vi "Main Page.vi"(8 "error in (no error)":errorcluster, 11 "Node Ptr":T6 format="%.0x") -> (0 "error out":errorcluster)   [LabVIEW 2021, in "Modbus Master System Explorer.lvlib"]
uses:
  Modbus Master System Explorer.lvlib
  <vilib>/NI VeriStand/Custom Device API/Custom Device Item Ref.ctl
  Shared/Controls/Interface Type.ctl
  Shared/Controls/Parity.ctl
  Shared/Controls/Serial Type.ctl
  Shared/Controls/Flow Control.ctl
  Shared/Write Mode.ctl
  Shared/Constants.vi
  <vilib>/NI VeriStand/Custom Device API/Set Item Property (U16).vi
  <vilib>/NI VeriStand/Custom Device API/Custom Device API.lvlib
  Shared/Modbus Master Shared.lvlib
panel:
  in  "Write Refresh Rate (ms)":i32
  in  "Write Mode":T1
  in  "WebBrowser":refnum<k7>(container)
  in  "Maximum Channels per Read":i32
  in  "Read Refresh Rate (ms)":i32
  in  "Export to Kepware Server":bool
  in  "Name":string
  in  "Master Settings Tabs":enum32{"TCP Master", "Serial Master"}(tab)
  in  "Timeout (ms)":i32
  in  "Address":string
  in  "Port":u16
  in  "Baud Rate":string(combo)
  out "Data Bits":u32=7
  in  "VISA resource name":refnum<visa-resource-name>
  in  "flow control (none)":T2 items=["None", "XON/XOFF", "RTS/CTS", "XON/XOFF & RTS/CTS", "DTR/DSR", "XON/XOFF & DTR/DSR"]
  in  "parity (even)":T3=2 items=["None", "Odd", "Even", "Mark", "Space"]
  in  "serial type":T4
  out "Stop Bits":u32
  in  "Wire Mode":i16(ring)=-2 items=["Non-NI RS485"=-2, "Unknown"=-1, "RS485/Wire4"=0, "RS485/Wire2-EchoDTR"=1, "RS485/Wire2-CtrlDTR"=2, "RS485/Wire2-Auto"=3, "RS232/DTE"=128, "RS232/DCE"=129, "RS232/AUTO"=130]
  in  "Interface Type":T5
  in  "Header":cluster{"Section Name":string}={"Section Name"="Modbus Master to Slave Settings"}
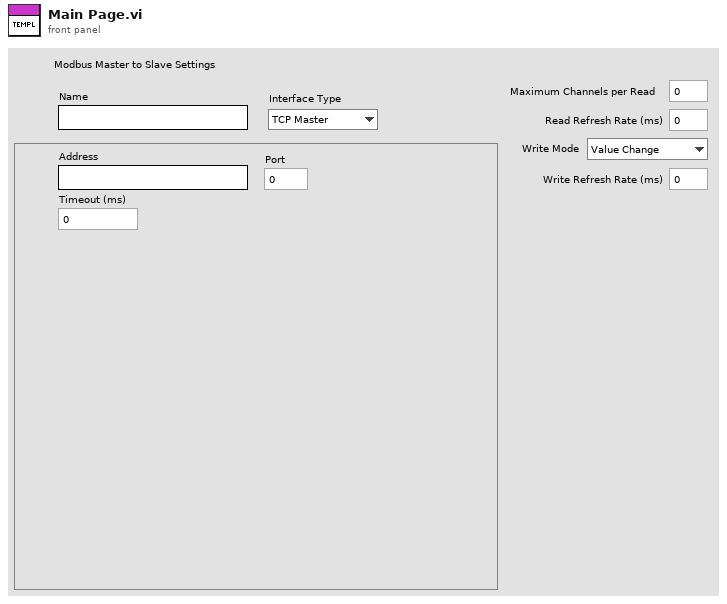
[diagram p1: front panel]
types:
  T1 = typedef "Modbus Master Shared.lvlib/Write Mode.ctl" = enum16{"Value Change", "Interval"}
  T2 = typedef "Modbus Master Shared.lvlib/Flow Control.ctl" = u16
  T3 = typedef "Modbus Master Shared.lvlib/Parity.ctl" = u16
  T4 = typedef "Modbus Master Shared.lvlib/Serial Type.ctl" = enum16{"RTU", "ASCII"}
  T5 = typedef "Modbus Master Shared.lvlib/Interface Type.ctl" = enum16{"TCP Master", "Serial Master", "TCP Slave", "Serial Slave"}
  T6 = typedef "Custom Device API.lvlib/Custom Device Item Ref.ctl" = u64
  T7 = enum8{"Enabled", "Disabled", "Disabled and Grayed Out"}
  T8 = typedef "Custom Device API.lvlib/Custom Device Commands.ctl" = enum16{"Default", "Item renamed", "Shutdown", "Dynamic button pressed"}
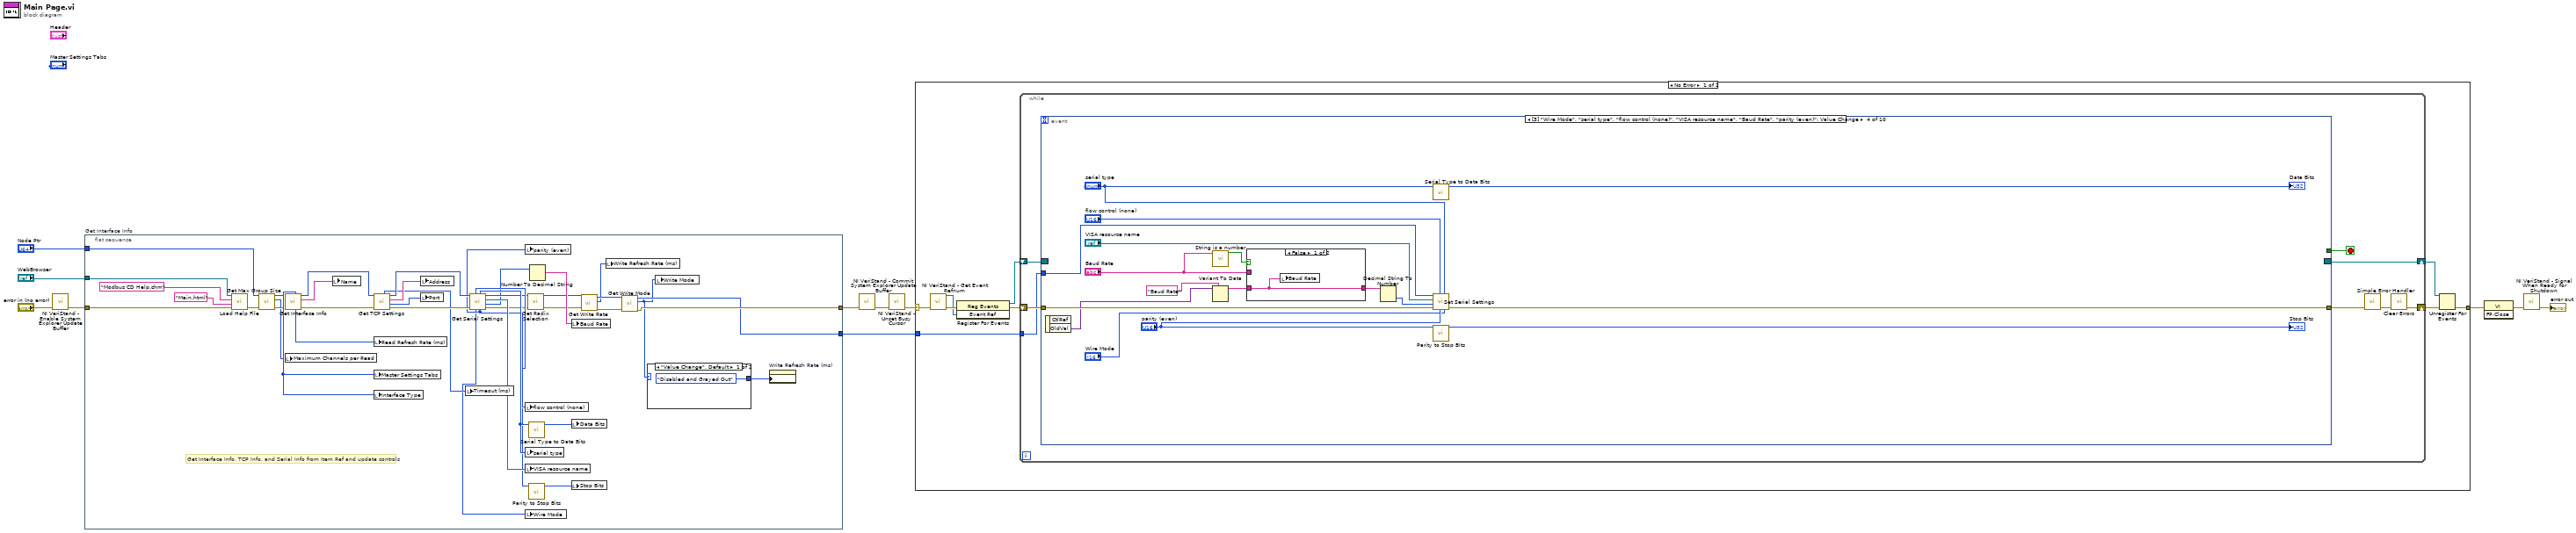
[diagram p0: block diagram]
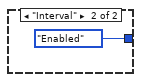
[diagram p2: hidden frame]
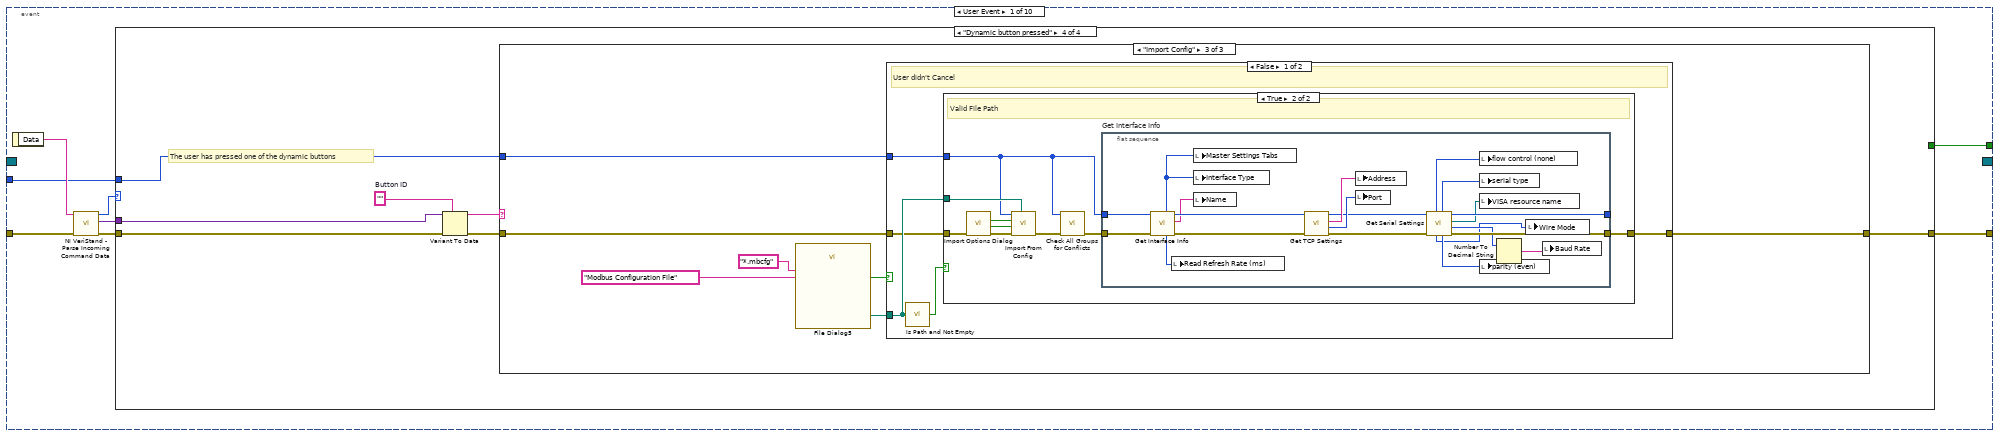
[diagram p3: hidden frame]
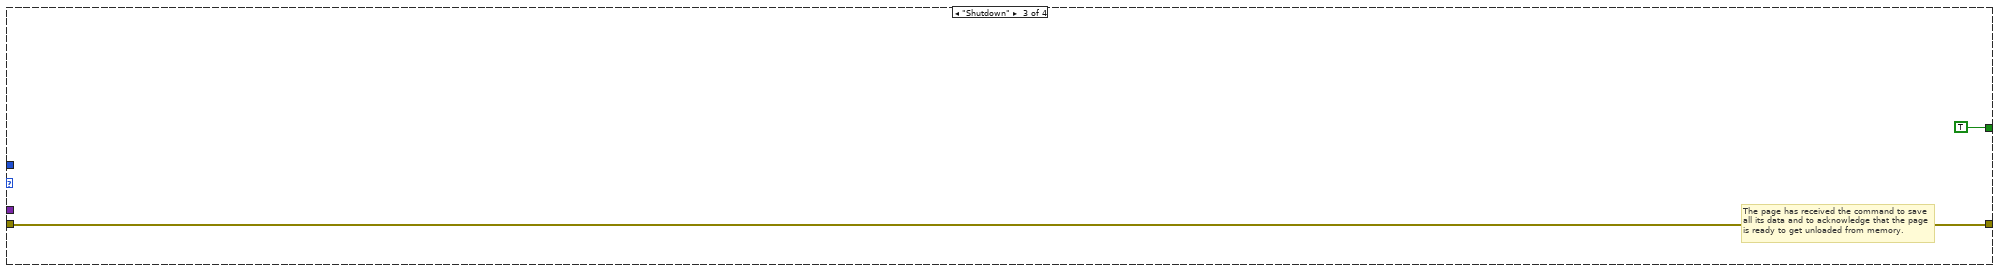
[diagram p6: hidden frame]
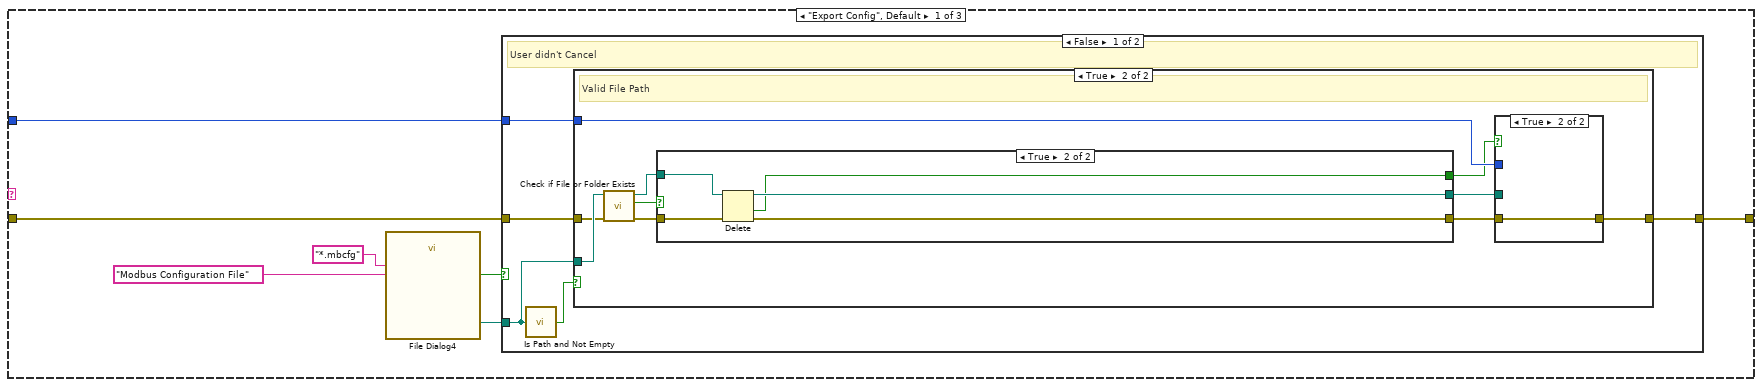
[diagram p7: hidden frame]
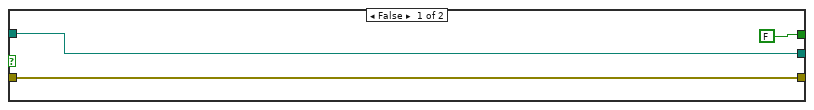
[diagram p9: hidden frame]
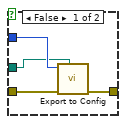
[diagram p10: hidden frame]
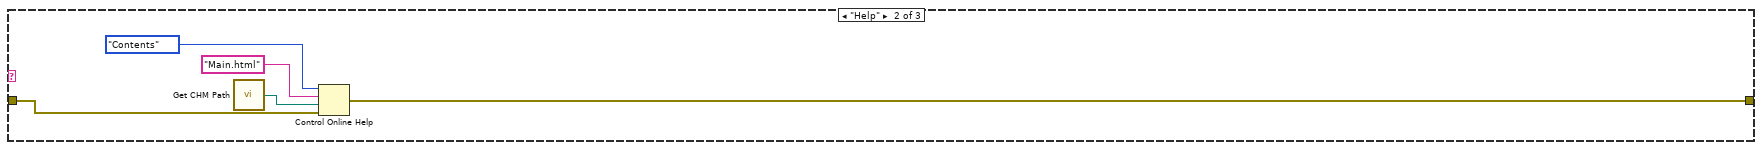
[diagram p12: hidden frame]
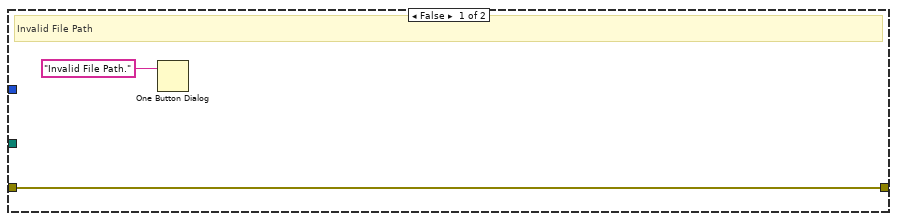
[diagram p13: hidden frame]
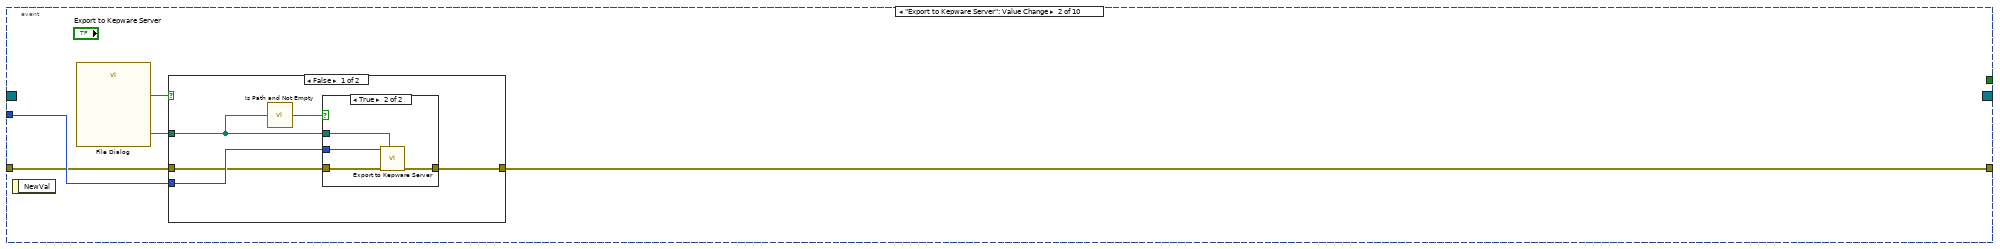
[diagram p15: hidden frame]
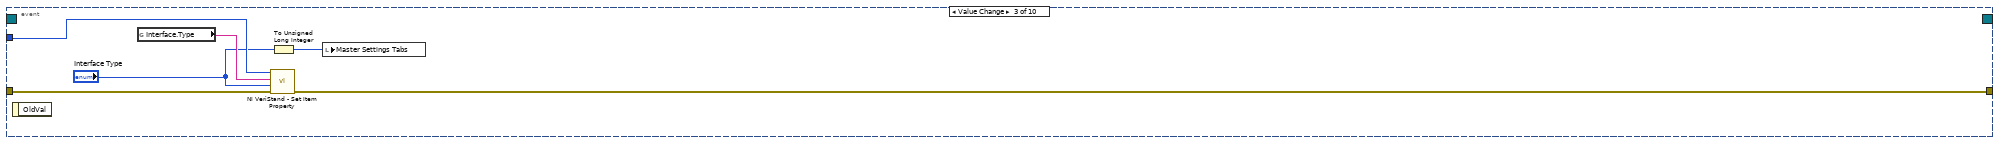
[diagram p18: hidden frame]
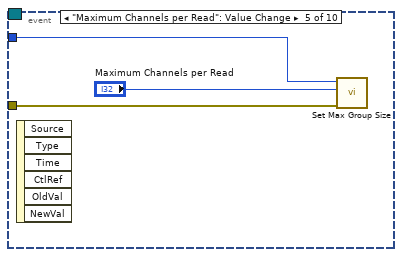
[diagram p20: hidden frame]
diagram:
  n1 = call <vilib>:"NI VeriStand - Enable System Explorer Update Buffer.vi"("error in (no error)"="error in (no error)") -> ("error out"=w1:errorcluster)  [unwired: 10 in]
  n2 = flat-sequence "Get Interface Info" {
    tunnel: w1 -> [w23]
    tunnel: "Node Ptr" -> [w35]
    tunnel: [w18] -> w4
    tunnel: [w15] -> w6
    tunnel: "WebBrowser" -> [w26]
    frame #0 {
      # "Get Interface Info, TCP Info, and Serial Info from Item Ref and update controls"
      n3 = call "Load Help File.vi"("error in (no error)"=w23, "HTML File"="Main.html", "Main CHM File"="Modbus CD Help.chm", "SHDocVw.IWebBrowser2"=w26) -> ("error out"=w22:errorcluster)  [unwired: 7 in]
      n4 = call "Get Max Group Size.vi"("error in (no error)"=w22, "Item Ref in"=w35) -> ("error out"=w33:errorcluster, "Value"=w32:i32, "Item Ref out"=w34:T6)  [unwired: 7 in]
      n5 = local write "Maximum Channels per Read"(w32) -> ()
      n6 = call "Get Interface Info.vi"("error in (no error)"=w33, "Device Item Ref in"=w34) -> ("error out"=w43:errorcluster, "Name"=w41:string, "Item Ref out"=w44:T6, "Refresh Rate"=w40:i32, "Interface Type"=w42:T5)  [unwired: 4 in, 1 out]
      n7 = local write "Name"(w41) -> ()
      n8 = call "Get TCP Settings.vi"("error in (no error)"=w43, "Item Ref in"=w44) -> ("error out"=w48:errorcluster, "Port"=w49:u16, "Address"=w50:string, "Item Ref out"=w47:T6, "Timeout"=w31:i32)  [unwired: 5 in]
      n9 = local write "Read Refresh Rate (ms)"(w40) -> ()
      n10 = local write "Master Settings Tabs"(w42) -> ()
      n11 = local write "Interface Type"(w42) -> ()
      n12 = local write "Address"(w50) -> ()
      n13 = local write "Port"(w49) -> ()
      n14 = local write "Timeout (ms)"(w31) -> ()
      n15 = call "Get Serial Settings.vi"("error in (no error)"=w48, "Item Ref in"=w47) -> ("error out"=w30:errorcluster, "baud rate"=w28:u32, "VISA resource name"=w45:refnum<visa-resource-name>, "Item Ref out"=w29:T6, "parity (even)"=w37:T3, "serial type"=w38:T4, "Wire Mode"=w21:i32, "flow control (none)"=w46:T2)  [unwired: 2 in]
      n16 = local write "parity (even)"(w37) -> ()
      n17 = local write "flow control (none)"(w46) -> ()
      n18 = local write "serial type"(w38) -> ()
      n19 = local write "VISA resource name"(w45) -> ()
      n20 = local write "Wire Mode"(w21) -> ()
      n21 = call "Get Radix Selection.vi"("error in (no error)"=w30, "Item Ref in"=w29) -> ("error out"=w20:errorcluster, "Item Ref out"=w17:T6)  [unwired: 7 in, 1 out]
      n22 = call "Serial Type to Data Bits.vi"("serial type"=w38) -> ("Data Bits"=w39:u32)  [unwired: 10 in]
      n23 = call "Parity to Stop Bits.vi"("parity"=w37) -> ("Stop Bits"=w36:u32)  [unwired: 10 in]
      n24 = Number To Decimal String(number=w28) -> (decimal integer string=w27:string)  [unwired: 1 in]
      n25 = local write "Baud Rate"(w27) -> ()
      n26 = local write "Data Bits"(w39) -> ()
      n27 = local write "Stop Bits"(w36) -> ()
      n28 = call "Get Write Rate.vi"("error in (no error)"=w20, "Item Ref in"=w17) -> ("error out"=w19:errorcluster, "Value"=w14:i32, "Item Ref out"=w16:T6)  [unwired: 7 in]
      n29 = local write "Write Refresh Rate (ms)"(w14) -> ()
      n30 = call "Get Write Mode.vi"("error in (no error)"=w19, "Item Ref in"=w16) -> ("error out"=w18:errorcluster, "Write Mode"=w12:T1, "Item Ref out"=w15:T6)  [unwired: 7 in]
      n31 = case shown="\"Value Change\", Default" w12 {
        tunnel: [T7."Disabled and Grayed Out" ("Disabled") T7."Enabled" ("Disabled")] -> w13
        frame "Value Change", Default {
        }
        frame "Interval" {
        }
      }
      n32 = local write "Write Mode"(w12) -> ()
      n33 = property on="Write Refresh Rate (ms)" class="DigNum (strict)"("DisabledEnum"=w13) -> ()  [unwired: 2 in, 2 out]
    }
  }
  n34 = call <vilib>:"NI VeriStand - Commit System Explorer Update Buffer.vi"("error in (no error)"=w4) -> ("error out"=w3:errorcluster)  [unwired: 10 in]
  n35 = call <vilib>:"NI VeriStand - Unset Busy Cursor.vi"("error in (no error)"=w3) -> ("error out"=w7:errorcluster)  [unwired: 10 out]
  n36 = case shown="No Error" w7 {
    selector: w7 -> [w53 w256]
    tunnel: [w58 w254] -> w11
    tunnel: w6 -> [w54 _]
    frame No Error {
      n37 = call <vilib>:"NI VeriStand - Get Event Refnum.vi"("error in (no error)"=w53) -> ("error out"=w61:errorcluster, "Event Ref"=w57:refnum<user-event>)  [unwired: 9 out]
      n38 = register-events(error in=w61, w57) -> (reference out=w55:refnum<event-registration>, error out=w56:errorcluster)  [unwired: 1 in]
      n39 = while {
        tunnel: w54 -> [w65]
        shift-right: [w62] -> w59
        shift-left: w56 -> [w68]
        shift-right: [w69] -> w60
        shift-left: w55 -> [w67]
        stop <- w66 stop-if-true
        n40 = event shown="[3] \"Wire Mode\", \"serial type\", \"flow control (none)\", \"VISA resource name\", \"Baud Rate\", \"parity (even)\": Value Change" {
          selector: w67 -> [_ _ _ _ _ _ _ _ _ _]
          dyn-events: [_ _ _ _ _ _ _ _ _ _] -> w69
          timeout: _ -> [_ _ _ _ _ _ _ _ _ _]
          tunnel: w68 -> [w77 w176 w194 w211 w216 w220 w225 w230 w234 w241]
          tunnel: [w73 _ _ _ _ _ _ _ _ _] -> w66
          tunnel: [w72 w175 w191 w209 _ w219 _ _ w233 w240] -> w64
          tunnel: w65 -> [w71 w177 w195 w212 w218 w222 w226 w231 w235 w242]
          event User Event {
            n41 = event-data() -> ("Data"=w76:string)  [unwired: 1 out]
            n42 = call <vilib>:"NI VeriStand - Parse Incoming Command Data.vi"("error in (no error)"=w77, "Incoming data"=w76) -> ("error out"=w75:errorcluster, "Outgoing data"=w70:variant, "Action"=w74:T8)  [unwired: 7 out]
            n43 = case shown="\"Dynamic button pressed\"" w74 {
              tunnel: w75 -> [w78 w79 w80 w88]
              tunnel: [_ _ TRUE _] -> w73
              tunnel: [w78 w79 w80 w82] -> w72
              tunnel: w71 -> [_ _ _ w84]
              tunnel: w70 -> [_ _ _ w87]
              frame "Default", Default {
              }
              frame "Item renamed" {
              }
              frame "Shutdown" {
                # "The page has received the command to save all its data and to acknowledge that the page is ready to get unloaded from memory."
              }
              frame "Dynamic button pressed" {
                w86 = ""  # Button ID
                # "The user has pressed one of the dynamic buttons"
                n44 = Variant To Data(error in=w88, type=w86, Variant=w87) -> (data=w85:string, error out=w83:errorcluster)
                n45 = case shown="\"Import Config\"" w85 {
                  tunnel: w84 -> [w93 _ w135]
                  tunnel: w83 -> [w92 w127 w134]
                  tunnel: [w91 w126 w133] -> w82
                  frame "Export Config", Default {
                    n46 = call "File Dialog4"("pattern (all files)"="*.mbcfg", "pattern label"="Modbus Configuration File") -> ("selected path"=w95:path, "cancelled"=w94:bool)  [unwired: 10 in, 2 out]
                    n47 = case shown="False" w94 {
                      tunnel: w95 -> [w99 _]
                      tunnel: w93 -> [w98 _]
                      tunnel: w92 -> [w97 w125]
                      tunnel: [w96 w125] -> w91
                      frame False {
                        # "User didn't Cancel"
                        n48 = call <vilib>:"Is Path and Not Empty.vi"("path"=w99) -> ("Is Path and Not Empty?"=w100:bool)  [unwired: 4 in]
                        n49 = case shown="True" w100 {
                          tunnel: w99 -> [_ w106]
                          tunnel: w98 -> [_ w110]
                          tunnel: w97 -> [w101 w103]
                          tunnel: [w101 w111] -> w96
                          frame False {
                          }
                          frame True {
                            # "Valid File Path"
                            n50 = call <vilib>:"Check if File or Folder Exists.vi"("error in (no error)"=w103, "path"=w106) -> ("error out"=w102:errorcluster, "file or folder exists?"=w104:bool, "dup path"=w105:path)  [unwired: 7 in]
                            n51 = case shown="True" w104 {
                              tunnel: [w114 w119] -> w109
                              tunnel: [FALSE ("cancelled") w118] -> w108
                              tunnel: w102 -> [w113 w117]
                              tunnel: [w113 w116] -> w107
                              tunnel: w105 -> [w114 w115]
                              frame False {
                              }
                              frame True {
                                n52 = Delete(path (use dialog)=w115, error in=w117) -> (deleted path=w119:path, cancelled=w118:bool, error out=w116:errorcluster)  [unwired: 3 in]
                              }
                            }
                            n53 = case shown="True" w108 {
                              tunnel: w107 -> [w123 w124]
                              tunnel: [w122 w124] -> w111
                              tunnel: w110 -> [w121 _]
                              tunnel: w109 -> [w120 _]
                              frame False {
                                n54 = call "Export to Config.vi"("selected path"=w120, "error in"=w123, "Device Ref in"=w121) -> ("error out"=w122:errorcluster)  [unwired: 8 in]
                              }
                              frame True {
                              }
                            }
                          }
                        }
                      }
                      frame True {
                      }
                    }
                  }
                  frame "Help" {
                    n55 = call "Get CHM Path.vi"() -> ("appended path"=w130:path)
                    n56 = Control Online Help(1:w127, 2:w130, 3:"Main.html" ("String to search for"), 4:enum16{"Contents", "Key", "Close"}."Contents" ("Operation")) -> (0:w126:errorcluster)
                  }
                  frame "Import Config" {
                    n57 = call "File Dialog5"("pattern (all files)"="*.mbcfg", "pattern label"="Modbus Configuration File") -> ("selected path"=w137:path, "cancelled"=w136:bool)  [unwired: 10 in, 2 out]
                    n58 = case shown="False" w136 {
                      tunnel: w137 -> [w141 _]
                      tunnel: w135 -> [w140 _]
                      tunnel: w134 -> [w139 w174]
                      tunnel: [w138 w174] -> w133
                      frame False {
                        # "User didn't Cancel"
                        n59 = call <vilib>:"Is Path and Not Empty.vi"("path"=w141) -> ("Is Path and Not Empty?"=w142:bool)  [unwired: 4 in]
                        n60 = case shown="True" w142 {
                          tunnel: w141 -> [_ w153]
                          tunnel: w140 -> [_ w151]
                          tunnel: w139 -> [w144 w148]
                          tunnel: [w144 w149] -> w138
                          frame False {
                            # "Invalid File Path"
                            n61 = One Button Dialog(message="Invalid File Path.") -> ()  [unwired: 1 in, 1 out]
                          }
                          frame True {
                            # "Valid File Path"
                            n62 = call "Import Options Dialog.vi"("error in (no error)"=w148) -> ("error out"=w147:errorcluster, "Overwrite Existing Channels?"=w145:bool, "Overwrite Device Settings?"=w146:bool)  [unwired: 8 in]
                            n63 = call "Import From Config.vi"("selected path"=w153, "error in"=w147, "Overwrite Existing Channels?"=w145, "Overwrite Device Settings?"=w146, "Device Ref in"=w151) -> ("error out"=w152:errorcluster)  [unwired: 6 in]
                            n64 = call "Check All Groups for Conflicts.vi"("error in (no error)"=w152, "Item Ref in"=w151) -> ("error out"=w150:errorcluster)  [unwired: 9 in]
                            n65 = flat-sequence "Get Interface Info" {
                              tunnel: w150 -> [w157]
                              tunnel: w151 -> [w158]
                              tunnel: [w170] -> w149
                              tunnel: [w168] -> _
                              frame #0 {
                                n66 = call "Get Interface Info.vi"("error in (no error)"=w157, "Device Item Ref in"=w158) -> ("error out"=w162:errorcluster, "Name"=w160:string, "Item Ref out"=w163:T6, "Refresh Rate"=w159:i32, "Interface Type"=w161:T5)  [unwired: 4 in, 1 out]
                                n67 = local write "Read Refresh Rate (ms)"(w159) -> ()
                                n68 = local write "Master Settings Tabs"(w161) -> ()
                                n69 = local write "Interface Type"(w161) -> ()
                                n70 = local write "Name"(w160) -> ()
                                n71 = call "Get TCP Settings.vi"("error in (no error)"=w162, "Item Ref in"=w163) -> ("error out"=w171:errorcluster, "Port"=w172:u16, "Address"=w173:string, "Item Ref out"=w169:T6)  [unwired: 5 in, 1 out]
                                n72 = local write "Address"(w173) -> ()
                                n73 = local write "Port"(w172) -> ()
                                n74 = call "Get Serial Settings.vi"("error in (no error)"=w171, "Item Ref in"=w169) -> ("error out"=w170:errorcluster, "baud rate"=w156:u32, "VISA resource name"=w164:refnum<visa-resource-name>, "Item Ref out"=w168:T6, "parity (even)"=w167:T3, "serial type"=w166:T4, "Wire Mode"=w154:i32, "flow control (none)"=w165:T2)  [unwired: 2 in]
                                n75 = local write "flow control (none)"(w165) -> ()
                                n76 = local write "serial type"(w166) -> ()
                                n77 = local write "VISA resource name"(w164) -> ()
                                n78 = local write "parity (even)"(w167) -> ()
                                n79 = Number To Decimal String(number=w156) -> (decimal integer string=w155:string)  [unwired: 1 in]
                                n80 = local write "Wire Mode"(w154) -> ()
                                n81 = local write "Baud Rate"(w155) -> ()
                              }
                            }
                          }
                        }
                      }
                      frame True {
                        # "User Canecelled, do nothing"
                      }
                    }
                  }
                }
              }
            }
          }
          event "Export to Kepware Server": Value Change {
            n82 = event-data() -> ()  [unwired: 2 out]
            n83 = call "File Dialog"() -> ("selected path"=w179:path, "cancelled"=w178:bool)  [unwired: 12 in, 2 out]
            n84 = case shown="False" w178 {
              tunnel: w179 -> [w183 _]
              tunnel: w177 -> [w182 _]
              tunnel: w176 -> [w181 w190]
              tunnel: [w180 w190] -> w175
              frame False {
                n85 = call <vilib>:"Is Path and Not Empty.vi"("path"=w183) -> ("Is Path and Not Empty?"=w184:bool)  [unwired: 4 in]
                n86 = case shown="True" w184 {
                  tunnel: w183 -> [_ w189]
                  tunnel: w182 -> [_ w188]
                  tunnel: w181 -> [w185 w187]
                  tunnel: [w185 w186] -> w180
                  frame False {
                  }
                  frame True {
                    n87 = call "Export to Kepware Server.vi"("selected path"=w189, "error in"=w187, "Device Ref in"=w188) -> ("error out"=w186:errorcluster)  [unwired: 8 in]
                  }
                }
              }
              frame True {
              }
            }
          }
          event Value Change {
            n88 = event-data() -> ()  [unwired: 2 out]
            n89 = global read "Constants.vi" "Interface.Type"() -> (w196:string)
            n90 = call-poly <vilib>:"NI VeriStand - Set Item Property.vi"("error in (no error)"=w194, "Value"="Interface Type", "Property Name"=w196, "Item Ref in"=w195) -> ("error out"=w191:errorcluster)  [unwired: 5 in, 2 out]
            n91 = To Unsigned Long Integer(number="Interface Type") -> (unsigned 32bit integer=w193:u32)
            n92 = local write "Master Settings Tabs"(w193) -> ()
          }
          event "Wire Mode", "VISA resource name", "Baud Rate": Value Change {
            n93 = event-data() -> ("OldVal"=w199:variant)  [unwired: 2 out]
            n94 = Variant To Data(type="Baud Rate" ("y"), Variant=w199) -> (data=w198:string)  [unwired: 1 in, 1 out]
            n95 = call "String is a number.vi"("Baud Rate"="Baud Rate") -> ("Boolean"=w202:bool)  [unwired: 10 in]
            n96 = case shown="False" w202 {
              tunnel: "Baud Rate" -> [_ w215]
              tunnel: [w214 w215] -> w200
              tunnel: w198 -> [w214 _]
              frame False {
                n97 = local write "Baud Rate"(w214) -> ()
              }
              frame True {
              }
            }
            n98 = Decimal String To Number(string=w200) -> (number=w206:i32)  [unwired: 2 in, 1 out]
            n99 = call "Serial Type to Data Bits.vi"("serial type"="serial type") -> ("Data Bits"=→"Data Bits":u32)  [unwired: 10 in]
            n100 = call "Set Serial Settings.vi"("Wire Mode"="Wire Mode", "serial type"="serial type", "parity (even)"="parity (even)", "flow control (none)"="flow control (none)", "error in (no error)"=w211, "baud rate"=w206, "VISA resource name"="VISA resource name", "Item Ref in"=w212) -> ("error out"=w209:errorcluster)  [unwired: 2 in, 1 out]
            n101 = call "Parity to Stop Bits.vi"("parity"="parity (even)") -> ("Stop Bits"=→"Stop Bits":u32)  [unwired: 10 in]
          }
          event "Maximum Channels per Read": Value Change {
            n102 = event-data() -> ()  [unwired: 7 out]
            n103 = call "Set Max Group Size.vi"("error in (no error)"=w216, "Value"="Maximum Channels per Read", "Item Ref in"=w218) -> ()  [unwired: 7 in, 2 out]
          }
          event "Name": Value Change {
            n104 = event-data() -> ()  [unwired: 4 out]
            n105 = call "update name.vi"("error in (no error)"=w220, "Desired Alias"="Name", "Parent Ref in"=w222) -> ("error out"=w219:errorcluster)  [unwired: 7 in, 1 out]
          }
          event Value Change {
            n106 = event-data() -> ()  [unwired: 7 out]
            n107 = call "Set Write Mode.vi"("error in (no error)"=w225, "Write Mode"="Write Mode", "Item Ref in"=w226) -> ()  [unwired: 7 in, 2 out]
            n108 = case shown="\"Value Change\", Default" "Write Mode" {
              tunnel: [T7."Disabled and Grayed Out" ("Disabled") T7."Enabled" ("Disabled")] -> w223
              frame "Value Change", Default {
              }
              frame "Interval" {
              }
            }
            n109 = property on="Write Refresh Rate (ms)" class="DigNum (strict)"("DisabledEnum"=w223) -> ()  [unwired: 2 in, 2 out]
          }
          event "Write Refresh Rate (ms)": Value Change {
            n110 = event-data() -> ()  [unwired: 7 out]
            n111 = call "Set Write Rate.vi"("error in (no error)"=w230, "Value"="Write Refresh Rate (ms)", "Item Ref in"=w231) -> ()  [unwired: 7 in, 2 out]
          }
          event "Read Refresh Rate (ms)": Value Change {
            n112 = event-data() -> ()  [unwired: 5 out]
            n113 = call "Set Refresh Rate.vi"("error in (no error)"=w234, "Value"="Read Refresh Rate (ms)", "Item Ref in"=w235) -> ("error out"=w233:errorcluster)  [unwired: 7 in, 1 out]
          }
          event "Address", "Port", "Timeout (ms)": Value Change {
            n114 = event-data() -> ()  [unwired: 4 out]
            n115 = call "IP Address Validity Check.vi"("IP Address"="Address") -> ("IP Address Vaidity Check"=w236:bool)  [unwired: 10 in]
            n116 = case shown="False" w236 {
              tunnel: w242 -> [w246 w253]
              tunnel: w241 -> [w247 w252]
              tunnel: [w244 w251] -> w240
              tunnel: "Port" -> [_ w250]
              tunnel: "Timeout (ms)" -> [_ w249]
              tunnel: "Address" -> [_ w248]
              frame False {
                n117 = One Button Dialog(message="Invalid IP Address!") -> ()  [unwired: 1 in, 1 out]
                n118 = call "Get TCP Settings.vi"("error in (no error)"=w247, "Item Ref in"=w246) -> ("error out"=w244:errorcluster, "Address"=w243:string)  [unwired: 5 in, 3 out]
                n119 = local write "Address"(w243) -> ()
              }
              frame True {
                n120 = call "Set TCP Settings.vi"("Timeout"=w249, "error in (no error)"=w252, "Port"=w250, "Address"=w248, "Item Ref in"=w253) -> ("error out"=w251:errorcluster)  [unwired: 5 in, 1 out]
              }
            }
          }
        }
        n121 = call <vilib>:"Simple Error Handler.vi"("error in (no error)"=w64) -> ("error out"=w63:errorcluster)  [unwired: 1 in, 7 out]
        n122 = call <vilib>:"Clear Errors.vi"("error in (no error)"=w63) -> ("error out"=w62:errorcluster)  [unwired: 1 in, 5 out]
      }
      n123 = Unregister For Events(event registration refnum=w60, error in=w59) -> (error out=w58:errorcluster)
    }
    frame Error {
      n124 = call <vilib>:"Simple Error Handler.vi"("error in (no error)"=w256) -> ("error out"=w255:errorcluster)  [unwired: 1 in, 7 out]
      n125 = call <vilib>:"Clear Errors.vi"("error in (no error)"=w255) -> ("error out"=w254:errorcluster)  [unwired: 1 in, 5 out]
    }
  }
  n126 = invoke class="VI" method="FP.Close"(error in=w11) -> (error out=w10:errorcluster)  [unwired: 2 in, 2 out]
  n127 = call <vilib>:"NI VeriStand - Signal When Ready for Shutdown.vi"("error in (no error)"=w10) -> ("error out"=→"error out":errorcluster)  [unwired: 10 out]
